vi "Reading bridge string.vi"(8 "error in":errorcluster, 10 "Previous":string, 11 "VISA in":refnum<visa-resource-name>) -> (0 "error out":errorcluster, 1 "Remaining":string, 2 "Message":string, 3 "VISA out":refnum<visa-resource-name>, 5 "Length":u32=66)   [LabVIEW 2017, in "Andeen-Hagerling 2700.lvlib"]
uses:
  <instrlib>/Andeen-Hagerling 2700/Andeen-Hagerling 2700.lvlib
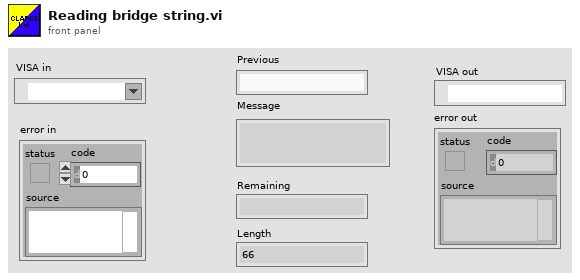
[diagram p1: front panel]
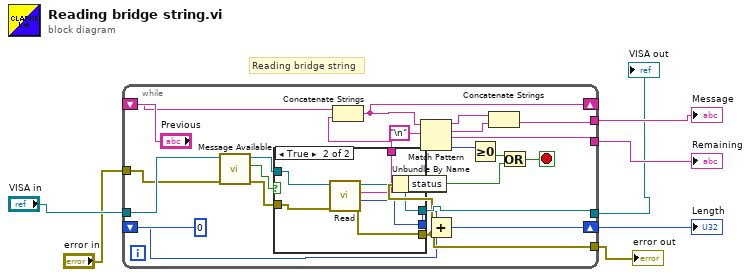
[diagram p0: block diagram]
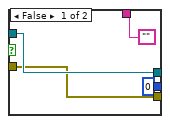
[diagram p2: hidden frame]
diagram:
  # "Reading bridge string"
  n1 = while {
    tunnel: [w28] -> w2
    tunnel: [w29] -> w1
    shift-right: [w26] -> w7
    shift-left: u32 0 -> [w25]
    shift-right: [w22] -> _
    shift-left: "Previous" -> [w23]
    tunnel: [w14] -> w8
    tunnel: [w13] -> w5
    tunnel: "VISA in" -> [w11]
    tunnel: "error in" -> [w10]
    stop <- w17 stop-if-true
    n2 = call <instrlib>:"Message Available.vi"("error in"=w10, "VISA resource name"=w11) -> ("error out"=w12:errorcluster, "message available"=w31:bool, "VISA resource name out"=w30:refnum<visa-resource-name>)  [unwired: 7 in]
    n3 = case shown="True" w31 {
      tunnel: w30 -> [w35 w41]
      tunnel: w12 -> [w34 w40]
      tunnel: [u32 0 ("Length") w39] -> w27
      tunnel: ["" w38] -> w24
      tunnel: [w35 w37] -> w29
      tunnel: [w34 w36] -> w28
      frame False {
      }
      frame True {
        n4 = call <instrlib>:"Read.vi"("error in"=w40, "VISA resource name"=w41) -> ("error out"=w36:errorcluster, "Length"=w39:u32, "Message"=w38:string, "VISA resource name out"=w37:refnum<visa-resource-name>)  [unwired: 6 in]
      }
    }
    n5 = Concatenate Strings(w23, w24) -> (w22:string)
    n6 = Unbundle By Name(w28) -> ("status"=w18:bool)
    n7 = Match Pattern(string=w22, regular expression="\n") -> (before substring=w16:string, match substring=w15:string, after substring=w14:string, offset past match=w20:i32)  [unwired: 1 in]
    n8 = Add(x=w25, y=w27) -> (x+y=w26:u32)
    n9 = Greater Or Equal To 0?(x=w20) -> (x >= 0?=w19:bool)
    n10 = Concatenate Strings(w16, w15) -> (w13:string)
    n11 = Or(x=w19, y=w18) -> (x .or. y?=w17:bool)
  }
  "Message" <- w5
  "Length" <- w7
  "Remaining" <- w8
  "error out" <- w2
  "VISA out" <- w1
